vi "OFDM RX - Simulated (No HW).vi"() -> ()   [LabVIEW 2012]
uses:
  <vilib>/Analysis/2dsp.llb/Complex FFT.vi
  <vilib>/addons/Modulation/Digital/General/MT Map QAM Symbols to Bits.vi
  <vilib>/Analysis/NI_AALPro.lvlib
  <vilib>/addons/Modulation/niDMT.lvlib
panel:
  out "Unequalized Data":cdb[](graph)
  out "Equalized Data":cdb[](graph)
  in  "Tab Control":enum32{"Parameters", "Debug", "CFO"}(tab)
  in  "IQ rate":dbl=5000000.0 format="%#_6p"
  in  "stop":bool
  out "Bit Error Rate":dbl format="%#_3g"
  out "output cluster":T1
  out "error out":errorcluster
  out "error out 2":errorcluster
  out "CFOest (Hz)":dbl[](array[numeric])
  out "theta":dbl[](graph)
  out "FFT {X}":dbl[](graph)
  out "Phase":dbl[](graph)
  out "Magnitude":dbl[](graph)
  # "OFDM Receiver - Simulation"
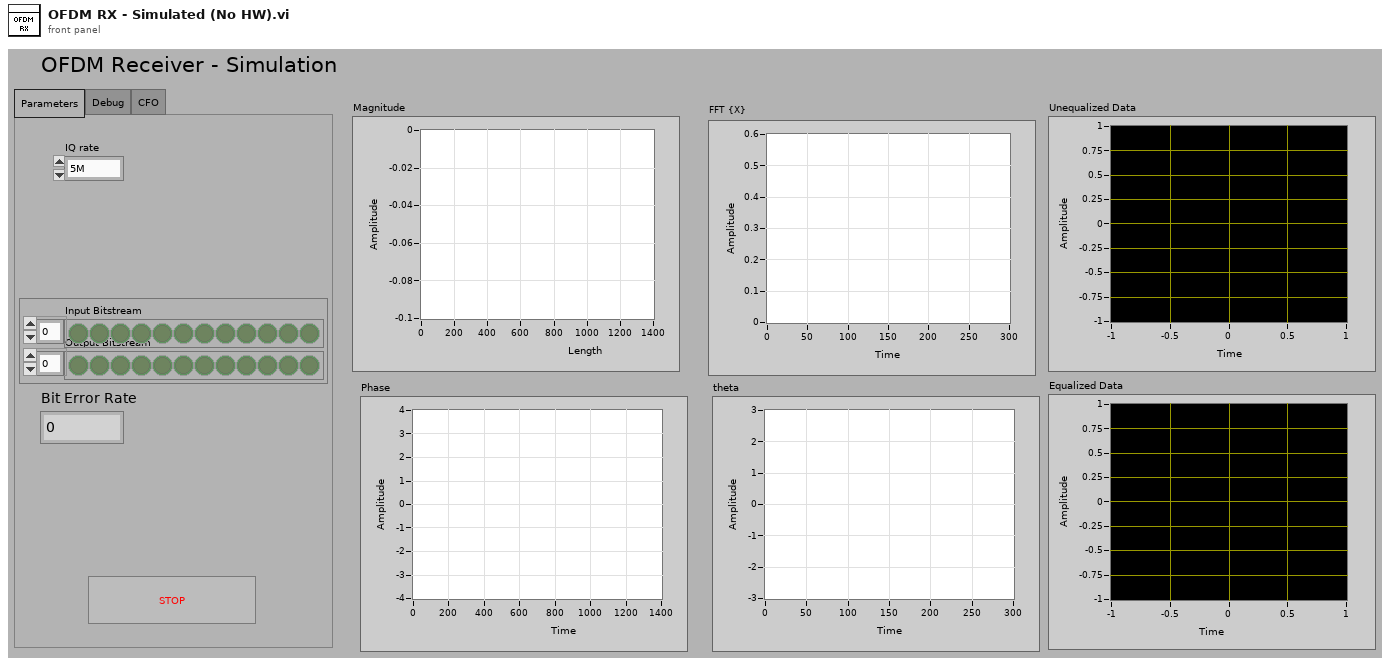
[diagram p1: front panel]
types:
  T1 = cluster{"Input Bitstream":bool[], "Output Bitstream":bool[]}
  T2 = cluster{"IQ Data":cdb[], "Original Bitstream":i8[]}
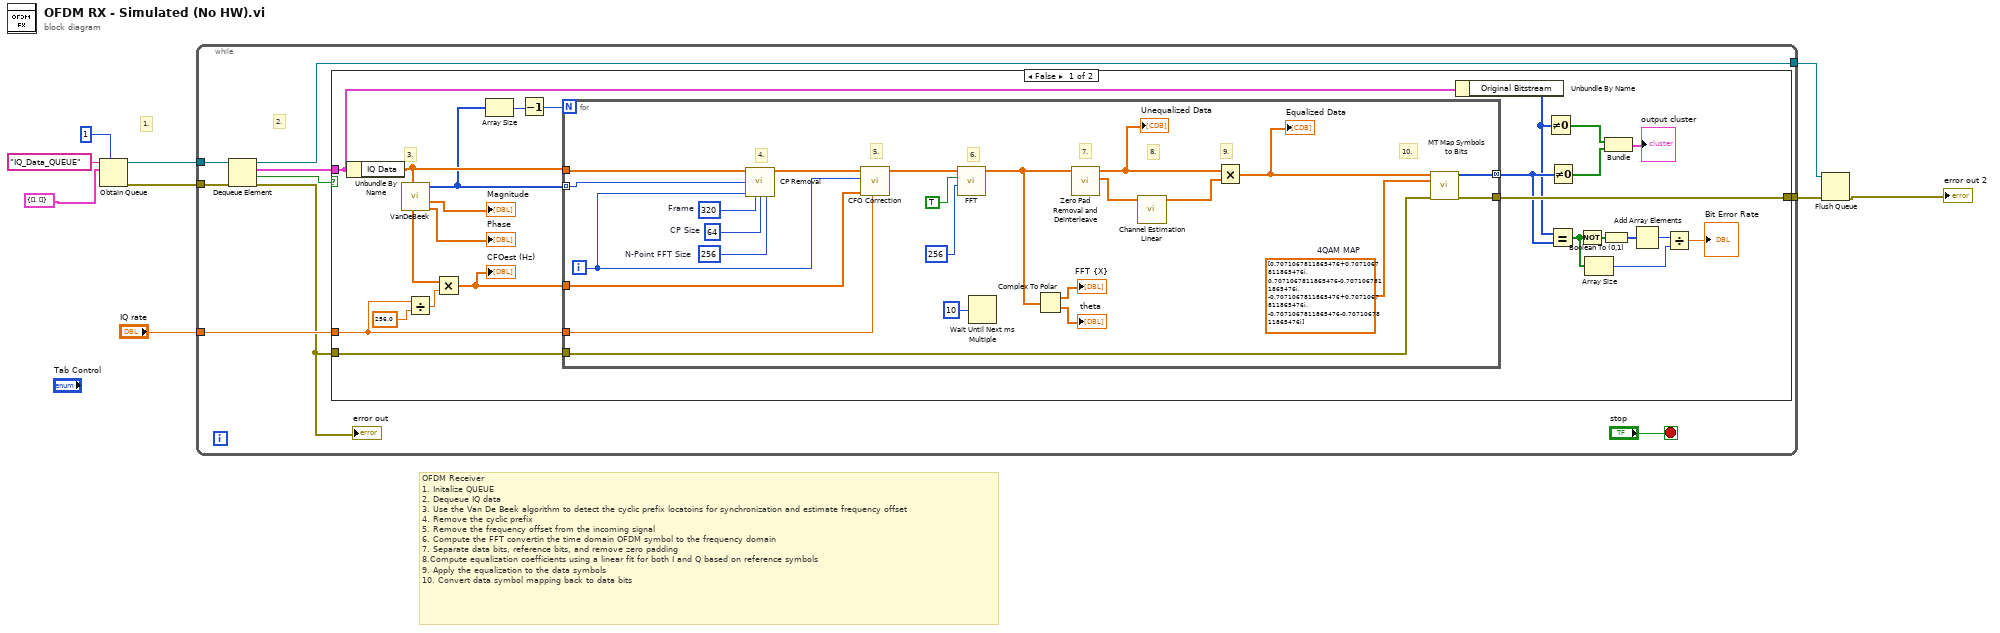
[diagram p0: block diagram]
diagram:
  # "1."
  # "OFDM Receiver\n1. Initalize QUEUE\n2. Dequeue IQ data\n3. Use the Van De Beek algorithm to detect the cyclic prefix locatoins for synchronization and estimate frequency offset\n4. Remove the cyclic prefix\n5. Remove the frequency offset from the incoming signal\n6. Compute the FFT convertin the time domain OFDM symbol to the frequency domain\n7. Separate data bits, reference bits, and remove zero padding\n8.Compute equalization coefficients using a linear fit for both I and Q based on reference symbols \n9. Apply the equalization to the data symbols\n10. Convert data symbol mapping back to data bits"
  n1 = Obtain Queue(max queue size (-1, unlimited)=1, name (unnamed)="IQ_Data_QUEUE", element data type=T2 {"IQ Data"=[], "Original Bitstream"=[]} ("output cluster")) -> (queue out=w6:refnum<queue>, error out=w5:errorcluster)  [unwired: 2 in, 1 out]
  n2 = while {
    tunnel: w6 -> [w15]
    tunnel: w5 -> [w14]
    tunnel: [w11] -> w2
    tunnel: "IQ rate" -> [w17]
    tunnel: [w16] -> w4
    stop <- "stop" stop-if-true
    # "2."
    n3 = Dequeue Element(queue=w15, error in (no error)=w14) -> (queue out=w11:refnum<queue>, element=w12:T2, timed out?=w10:bool, error out=w13:errorcluster)  [unwired: 1 in]
    "error out" <- w13
    n4 = case shown="False" w10 {
      tunnel: w17 -> [w43 _]
      tunnel: [w42 w68] -> w16
      tunnel: w13 -> [w35 w68]
      tunnel: w12 -> [w25 _]
      frame False {
        # "3."
        n5 = Unbundle By Name(w25) -> ("IQ Data"=w26:cdb[])
        n6 = call <userlib>:"VanDeBeek.vi"("Input"=w26) -> ("Phase"=→"Phase":dbl[], "Magnitude"=→"Magnitude":dbl[], "Indices"=w19:i32[], "CFOest (Hz)"=w39:dbl[])  [unwired: 6 in, 1 out]
        n7 = Divide(x=w43, y=256.0 ("x")) -> (x/y=w40:dbl)
        n8 = Multiply(x=w39, y=w40) -> (x*y=w36:dbl[])
        "CFOest (Hz)" <- w36
        n9 = Array Size(array=w19) -> (size(s)=w21:i32)
        n10 = Decrement(x=w21) -> (x-1=w20:i32)
        n11 = for {
          N: w20 -> [_]
          tunnel: w36 -> [w60]
          tunnel: w43 -> [w59]
          tunnel: w35 -> [w58]
          tunnel: [w57] -> w42
          tunnel: w19 -> [w52] mode=indexing
          tunnel: w26 -> [w55]
          tunnel: [w46] -> w28 mode=concatenating
          i -> [w50]
          w51 = 256  # N-Point FFT Size
          w54 = 64  # CP Size
          w61 = cdb[] [0.7071067811865476+0.7071067811865476i, 0.7071067811865476-0.7071067811865476i, -0.7071067811865476+0.7071067811865476i, -0.7071067811865476-0.7071067811865476i]  # 4QAM MAP
          w53 = 320  # Frame
          # "10."
          # "9."
          # "8."
          # "7."
          # "6."
          # "5."
          # "4."
          n12 = call <userlib>:"CP Removal.vi"("Input"=w55, "Indicies"=w52, "i"=w50, "Frame Size"=w53, "CP Size"=w54, "N-Point FFT Size"=w51) -> ("Output Without CP"=w56:cdb[])  [unwired: 9 in]
          n13 = call <userlib>:"CFO Correction.vi"("fs"=w59, "CFOest (freq)"=w60, "Index"=w50, "Input"=w56) -> ("Output"=w62:cdb[])  [unwired: 7 in]
          n14 = call-poly <vilib>:"FFT.vi"("FFT size"=256, "shift?"=TRUE, "X"=w62) -> ("FFT {X}"=w63:cdb[])  [unwired: 7 in, 1 out]
          n15 = Wait Until Next ms Multiple(millisecond multiple=u32 10) -> ()  [unwired: 1 out]
          n16 = Complex To Polar(r * e^(i*theta)=w63) -> (r=→"FFT {X}":dbl[], theta=→"theta":dbl[])
          n17 = call <userlib>:"Zero Pad Removal and Deinterleave.vi"("Input"=w63) -> ("Ref"=w48:cdb[], "Data"=w45:cdb[])  [unwired: 9 in]
          "Unequalized Data" <- w45
          n18 = call <userlib>:"Channel Estimation Linear.vi"("Ref"=w48) -> ("Hest"=w47:cdb[])  [unwired: 10 in]
          n19 = Multiply(x=w45, y=w47) -> (x*y=w44:cdb[])
          "Equalized Data" <- w44
          n20 = call-poly <vilib>:"MT Map Symbols to Bits.vi"("symbols"=w44, "symbol map"=w61, "error in (no error)"=w58) -> ("output bit stream"=w46:i8[], "error out"=w57:errorcluster)  [unwired: 11 in]
        }
        n21 = Unbundle By Name(w25) -> ("Original Bitstream"=w27:i8[])
        n22 = Not Equal To 0?(x=w27) -> (x != 0?=w24:bool[])
        n23 = Equal?(x=w27, y=w28) -> (x = y?=w34:bool[])
        n24 = Not Equal To 0?(x=w28) -> (x != 0?=w23:bool[])
        n25 = Not(x=w34) -> (.not. x?=w33:bool[])
        n26 = Array Size(array=w34) -> (size(s)=w30:i32)
        n27 = Boolean To (0,1)(Boolean=w33) -> (0, 1=w32:i16[])
        n28 = Bundle(w24, w23) -> (→"output cluster":cluster{bool[], bool[]})  [unwired: 1 in]
        n29 = Add Array Elements(numeric array=w32) -> (sum=w31:i16)
        n30 = Divide(x=w31, y=w30) -> (x/y=→"Bit Error Rate":dbl)
      }
      frame True {
      }
    }
  }
  n31 = Flush Queue(queue=w2, error in (no error)=w4) -> (error out=→"error out 2":errorcluster)  [unwired: 2 out]
